vi "Decompose Set.vi"(8 "error in (no error)":errorcluster, 11 "Variant Set":variant) -> (0 "error out":errorcluster, 2 "Elements":variant[](array[variant]), 3 "Size":i32)   [LabVIEW 2017, in "Composition.lvlib"]
doc: "Decomposes a Variant Set into Variant elements. Sets are available in LabVIEW 2019 and higher.\n\n<B>Important</B>\nThis VI is not safe to use in LabVIEW 2019 to 2023 Q3 because of a known issue in the Variant To Flattened String primitive. See LabVIEW issue number 2058864 for further information."
uses:
  Composition.lvlib
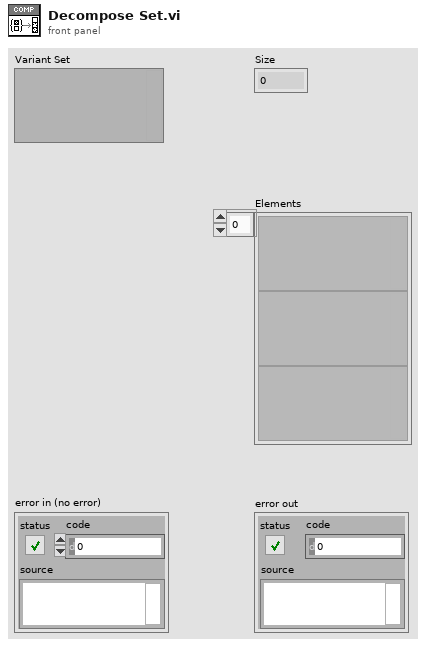
[diagram p1: front panel]
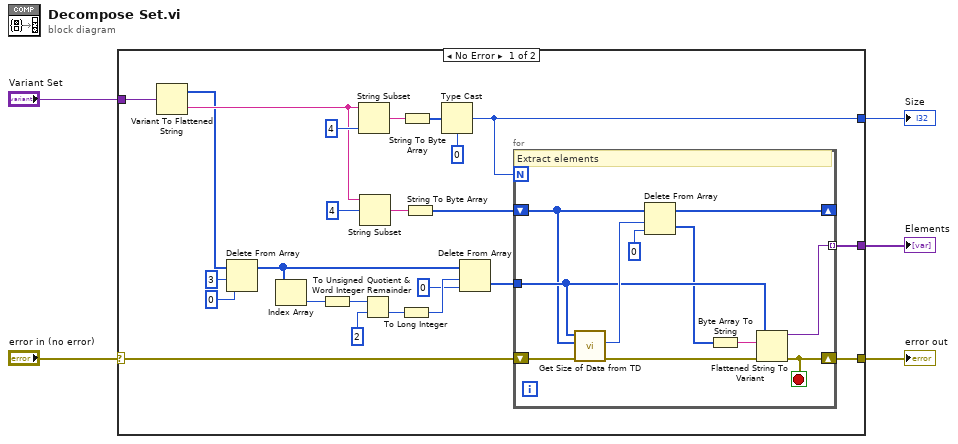
[diagram p0: block diagram]
diagram:
  n1 = case shown="No Error" "error in (no error)" {
    selector: "error in (no error)" -> [w19 w41]
    tunnel: [w22 _] -> w5
    tunnel: "Variant Set" -> [w21 _]
    tunnel: [w20 w41] -> w3
    tunnel: [w15 _] -> w2
    frame No Error {
      n2 = Variant To Flattened String(Variant=w21) -> (data string=w25:string, 1:w18:i16[])
      n3 = Delete From Array(array=w18, length=3, index=0) -> (array with subset deleted=w7:i16[])  [unwired: 1 out]
      n4 = Index Array(array=w7) -> (element=w13:i16)  [unwired: 1 in]
      n5 = To Unsigned Word Integer(number=w13) -> (unsigned 16bit integer=w11:u16)
      n6 = String Subset(string=w25, length (rest)=4 ("length (rest)")) -> (substring=w29:string)  [unwired: 1 in]
      n7 = String Subset(string=w25, offset (0)=4) -> (substring=w23:string)  [unwired: 1 in]
      n8 = Quotient & Remainder(x=w11, y=u16 2) -> (floor(x/y)=w10:u16)  [unwired: 1 out]
      n9 = To Long Integer(number=w10) -> (32bit integer=w9:i32)
      n10 = String To Byte Array(string=w29) -> (unsigned byte array=w26:u8[])
      n11 = String To Byte Array(string=w23) -> (unsigned byte array=w14:u8[])
      n12 = Type Cast(type=0, x=w26) -> (*(type *) &x=w15:i32)
      n13 = Delete From Array(array=w7, length=w9, index=0) -> (deleted portion=w6:i16[])  [unwired: 1 out]
      n14 = for {
        N: w15 -> [_]
        shift-right: [w37] -> _
        shift-left: w14 -> [w31]
        tunnel: [w40] -> w22 mode=indexing
        shift-right: [w38] -> w20
        shift-left: w19 -> [w35]
        tunnel: w6 -> [w32]
        stop <- w38 stop-if-true
        # "Extract elements"
        n15 = call "Get Size of Data from TD.vi"("error in (no error)"=w35, "Data String"=w31, "Type Descriptor"=w32) -> ("error out"=w34:errorcluster, "Size of Data"=w33:i32)  [unwired: 7 in]
        n16 = Delete From Array(array=w31, length=w33, index=0) -> (deleted portion=w30:u8[], array with subset deleted=w37:u8[])
        n17 = Byte Array To String(unsigned byte array=w30) -> (string=w39:string)
        n18 = Flattened String To Variant(4:w34, 6:w39, 7:w32) -> (0:w38:errorcluster, 3:w40:variant)
      }
    }
    frame Error {
    }
  }
  "Size" <- w2
  "Elements" <- w5
  "error out" <- w3
